vi "Button_handling.vi"(7 "connect":bool, 10 "Z_HSwitch":bool, 11 "Z_Source":T2=enum."local disabled") -> (3 "Z_HSwitch_state":T1={"Write"=FALSE, "Z1_ind"=5, "Z1_ind_blinking"=FALSE, "Z_HSwitch_out"=FALSE, "Z_HSwitch_visible"=FALSE, "Z_HSwitch_disabled"=enum."Enabled"})   [LabVIEW 2019]
uses:
  Y_source.ctl
  OLD/Button state.ctl
  Timer Delay/Timers.lvlib
panel:
  out "Z1 ind":u8(ring)
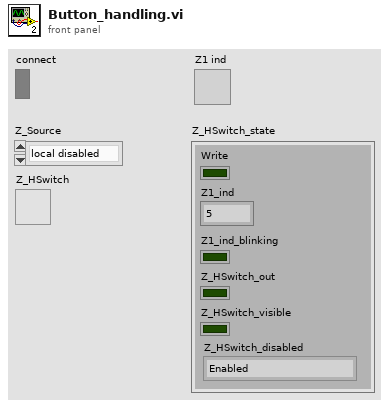
[diagram p1: front panel]
types:
  T1 = cluster{"Write":bool, "Z1_ind":u8, "Z1_ind_blinking":bool, "Z_HSwitch_out":bool, "Z_HSwitch_visible":bool, "Z_HSwitch_disabled":enum8{"Enabled", "Disabled", "Disabled and Grayed Out"}}
  T2 = typedef "Y_source.ctl" = enum8{"initialize", "local disabled", "local hand", "hand", "auto", "dist"}
  T3 = enum8{"Enabled", "Disabled", "Disabled and Grayed Out"}
  T4 = typedef "Button state.ctl" = enum16{"init", "not connect", "local disabled", "local hand", "set hand", "hand", "set auto", "auto", "dist"}
  T5 = cluster{"Write":bool, "Z1_ind visu":u8, "Z1_ind_blinking":bool, "Z_HSwitch_out":bool, "Z_HSwitch_visible":bool, "Z_HSwitch_disabled":enum8{"Enabled", "Disabled", "Disabled and Grayed Out"}}
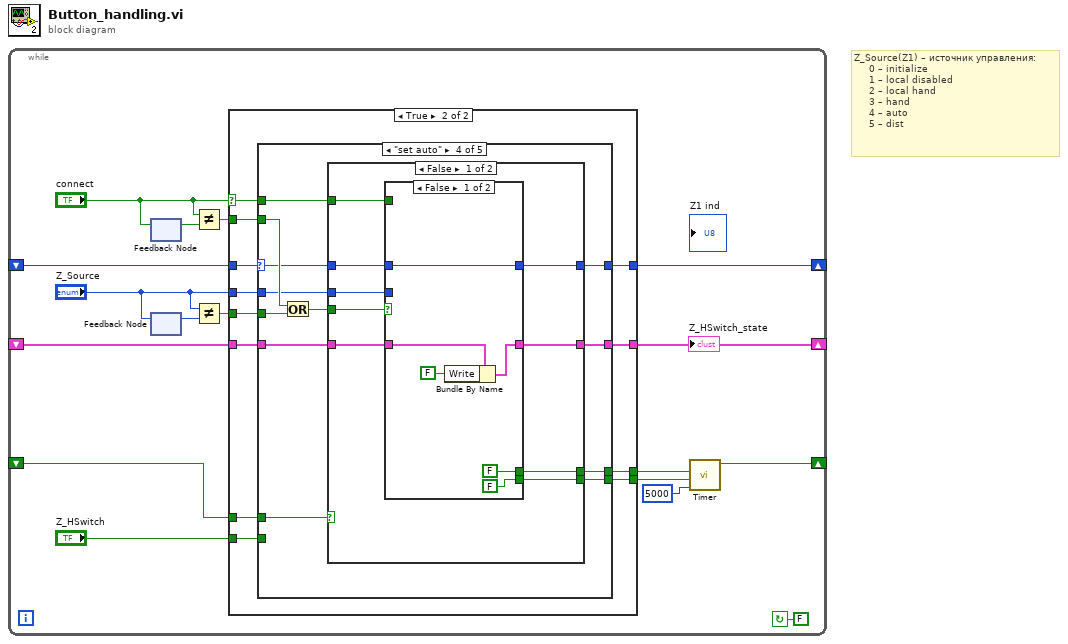
[diagram p0: block diagram]
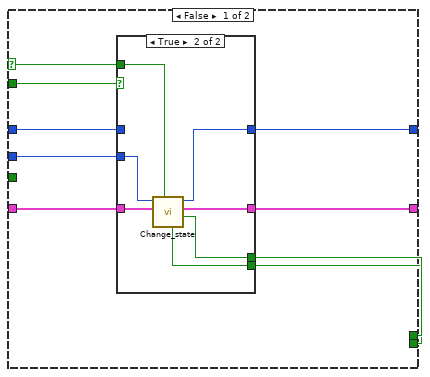
[diagram p2: hidden frame]
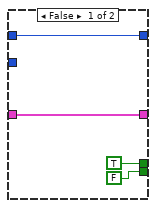
[diagram p3: hidden frame]
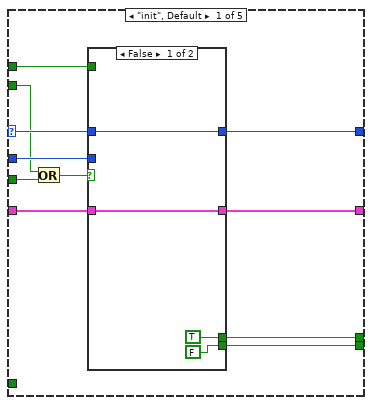
[diagram p4: hidden frame]
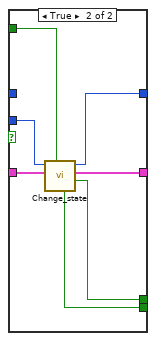
[diagram p5: hidden frame]
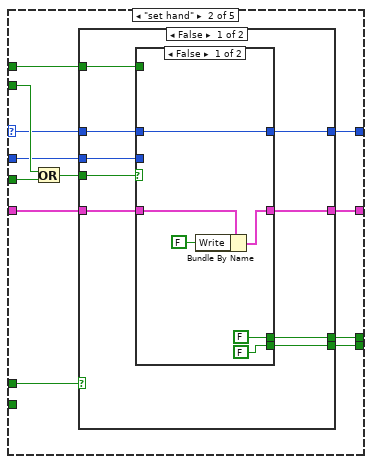
[diagram p6: hidden frame]
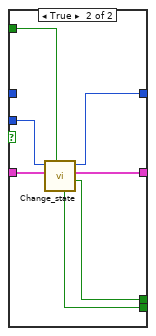
[diagram p7: hidden frame]
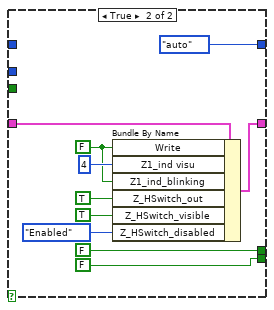
[diagram p8: hidden frame]
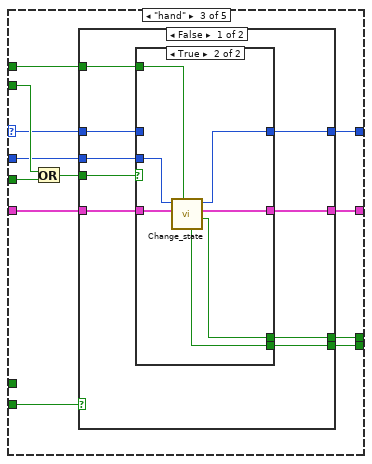
[diagram p9: hidden frame]
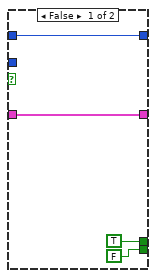
[diagram p10: hidden frame]
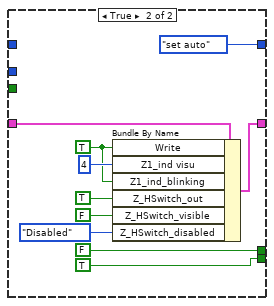
[diagram p11: hidden frame]
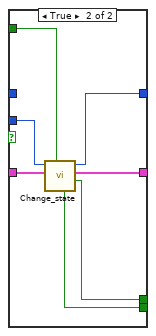
[diagram p12: hidden frame]
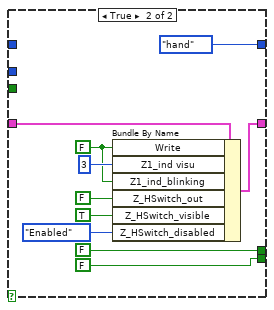
[diagram p13: hidden frame]
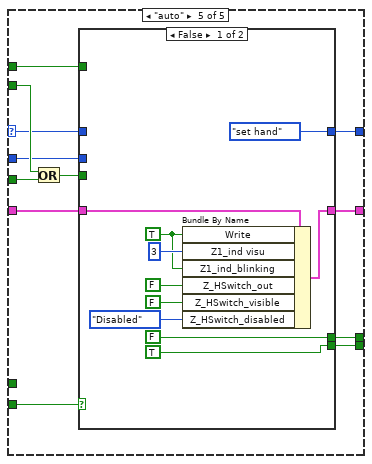
[diagram p14: hidden frame]
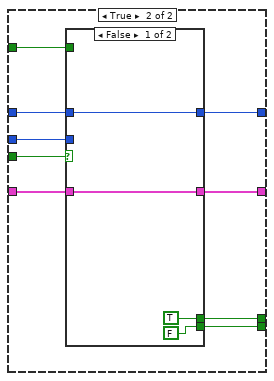
[diagram p15: hidden frame]
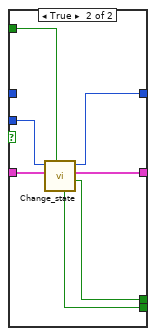
[diagram p16: hidden frame]
diagram:
  # "Z_Source(Z1) – источник управления:\n     0 – initialize\n     1 – local disabled\n     2 – local hand\n     3 – hand\n     4 – аuto\n     5 – dist"
  n1 = while {
    shift-right: [w17] -> _
    shift-left: _ -> [w1]
    shift-right: [w12] -> _
    shift-left: _ -> [w16]
    shift-right: [w10] -> _
    shift-left: _ -> [w13]
    stop <- FALSE continue-if-true
    n2 = feedback #1() -> (w4:bool)  [unwired: 1 in]
    n3 = feedback-in #1("connect") -> ()
    n4 = feedback #2() -> (w7:T2)  [unwired: 1 in]
    n5 = feedback-in #2("Z_Source") -> ()
    n6 = Not Equal?(x="connect", y=w4) -> (x != y?=w2:bool)
    n7 = Not Equal?(x="Z_Source", y=w7) -> (x != y?=w5:bool)
    n8 = case shown="True" "connect" {
      selector: "connect" -> [w18 w40]
      tunnel: [w23 w49] -> w17
      tunnel: w16 -> [_ w48]
      tunnel: w13 -> [w24 w47]
      tunnel: w1 -> [w26 w46]
      tunnel: "Z_HSwitch" -> [_ w45]
      tunnel: "Z_Source" -> [w25 w44]
      tunnel: [w22 w43] -> w10
      tunnel: [w21 w42] -> w9
      tunnel: [w20 w41] -> w8
      tunnel: w5 -> [_ w39]
      tunnel: w2 -> [w19 w38]
      frame False {
        n9 = case shown="True" w19 {
          tunnel: w24 -> [w30 w37]
          tunnel: [w30 w36] -> w22
          tunnel: [TRUE ("reset_timer") w35] -> w21
          tunnel: [FALSE ("load_timer") w34] -> w20
          tunnel: [w27 w33] -> w23
          tunnel: w25 -> [_ w32]
          tunnel: w26 -> [w27 _]
          tunnel: w18 -> [_ w31]
          frame False {
          }
          frame True {
            n10 = call "Change_state.vi"("connect (T)"=w31, "Z_HSwitch_state in"=w37, "Z_Source"=w32) -> ("reset_timer"=w35:bool, "Z_HSwitch_state out"=w36:T5, "Z1_ind_state"=w33:T4, "load_timer"=w34:bool)  [unwired: 5 in]
          }
        }
      }
      frame True {
        n11 = case shown="\"set auto\"" w46 {
          selector: w46 -> [w54 w75 w119 w161 w205]
          tunnel: w45 -> [_ _ w121 _ w207]
          tunnel: [w55 w81 w125 w167 w211] -> w49
          tunnel: w44 -> [w59 w74 w118 w160 w204]
          tunnel: w48 -> [_ w77 _ w163 _]
          tunnel: [w58 w79 w123 w165 w209] -> w42
          tunnel: [w57 w78 w122 w164 w208] -> w41
          tunnel: [w56 w80 w124 w166 w210] -> w43
          tunnel: w47 -> [w60 w72 w116 w158 w202]
          tunnel: w40 -> [w51 w76 w120 w162 w206]
          tunnel: w39 -> [w52 w82 w126 w168 w212]
          tunnel: w38 -> [w50 w83 w127 w169 w213]
          frame "init", Default {
            # "local hand"
            n12 = Or(x=w50, y=w52) -> (x .or. y?=w53:bool)
            n13 = case shown="False" w53 {
              tunnel: w60 -> [w64 w71]
              tunnel: [w64 w70] -> w56
              tunnel: [TRUE ("reset_timer") w69] -> w58
              tunnel: [FALSE ("load_timer") w68] -> w57
              tunnel: [w61 w67] -> w55
              tunnel: w59 -> [_ w66]
              tunnel: w51 -> [_ w65]
              tunnel: w54 -> [w61 _]
              frame False {
              }
              frame True {
                n14 = call "Change_state.vi"("connect (T)"=w65, "Z_HSwitch_state in"=w71, "Z_Source"=w66) -> ("reset_timer"=w69:bool, "Z_HSwitch_state out"=w70:T5, "Z1_ind_state"=w67:T4, "load_timer"=w68:bool)  [unwired: 5 in]
              }
            }
          }
          frame "set hand" {
            # "local hand"
            n15 = Or(x=w83, y=w82) -> (x .or. y?=w73:bool)
            n16 = case shown="False" w77 {
              tunnel: w75 -> [w87 _]
              tunnel: [w86 Button_state."auto" ("f 3")] -> w81
              tunnel: [w84 w110] -> w80
              tunnel: w72 -> [w85 w109]
              tunnel: [w89 FALSE ("Z_ASwitch")] -> w79
              tunnel: [w88 FALSE ("Z_ASwitch")] -> w78
              tunnel: w76 -> [w92 _]
              tunnel: w74 -> [w91 _]
              tunnel: w73 -> [w90 _]
              frame False {
                n17 = case shown="False" w90 {
                  tunnel: w85 -> [w94 w105]
                  tunnel: [w93 w104] -> w84
                  tunnel: [FALSE ("reset_timer") w103] -> w89
                  tunnel: [FALSE ("load_timer") w102] -> w88
                  tunnel: [w96 w101] -> w86
                  tunnel: w91 -> [_ w100]
                  tunnel: w92 -> [_ w99]
                  tunnel: w87 -> [w96 _]
                  frame False {
                    n18 = Bundle By Name(cluster=w94, "Write"=FALSE) -> (w93:T5)
                  }
                  frame True {
                    n19 = call "Change_state.vi"("connect (T)"=w99, "Z_HSwitch_state in"=w105, "Z_Source"=w100) -> ("reset_timer"=w103:bool, "Z_HSwitch_state out"=w104:T5, "Z1_ind_state"=w101:T4, "load_timer"=w102:bool)  [unwired: 5 in]
                  }
                }
              }
              frame True {
                w112 = FALSE ("Z_ASwitch")
                n20 = Bundle By Name(cluster=w109, "Write"=w112, "Z1_ind visu"=u8 4, "Z1_ind_blinking"=w112, "Z_HSwitch_out"=TRUE ("Z_ASwitch"), "Z_HSwitch_visible"=TRUE ("Z_ASwitch"), "Z_HSwitch_disabled"=T3."Enabled" ("Disabled")) -> (w110:T5)
              }
            }
          }
          frame "hand" {
            # "local hand"
            n21 = Or(x=w127, y=w126) -> (x .or. y?=w117:bool)
            n22 = case shown="False" w121 {
              tunnel: w119 -> [w129 _]
              tunnel: [w128 Button_state."set auto" ("f 3")] -> w125
              tunnel: [w130 w152] -> w124
              tunnel: w116 -> [w131 w151]
              tunnel: [w133 FALSE ("Z_ASwitch")] -> w123
              tunnel: [w132 TRUE ("Z_ASwitch")] -> w122
              tunnel: w120 -> [w136 _]
              tunnel: w118 -> [w135 _]
              tunnel: w117 -> [w134 _]
              frame False {
                n23 = case shown="True" w134 {
                  tunnel: w131 -> [w140 w147]
                  tunnel: [w140 w146] -> w130
                  tunnel: [TRUE ("reset_timer") w145] -> w133
                  tunnel: [FALSE ("load_timer") w144] -> w132
                  tunnel: [w137 w143] -> w128
                  tunnel: w135 -> [_ w142]
                  tunnel: w136 -> [_ w141]
                  tunnel: w129 -> [w137 _]
                  frame False {
                  }
                  frame True {
                    n24 = call "Change_state.vi"("connect (T)"=w141, "Z_HSwitch_state in"=w147, "Z_Source"=w142) -> ("reset_timer"=w145:bool, "Z_HSwitch_state out"=w146:T5, "Z1_ind_state"=w143:T4, "load_timer"=w144:bool)  [unwired: 5 in]
                  }
                }
              }
              frame True {
                w154 = TRUE ("Z_ASwitch")
                n25 = Bundle By Name(cluster=w151, "Write"=w154, "Z1_ind visu"=u8 4, "Z1_ind_blinking"=w154, "Z_HSwitch_out"=TRUE ("Z_ASwitch"), "Z_HSwitch_visible"=FALSE ("Z_ASwitch"), "Z_HSwitch_disabled"=T3."Disabled" ("Disabled")) -> (w152:T5)
              }
            }
          }
          frame "set auto" {
            # "local hand"
            n26 = Or(x=w169, y=w168) -> (x .or. y?=w159:bool)
            n27 = case shown="False" w163 {
              tunnel: w161 -> [w173 _]
              tunnel: [w172 Button_state."hand" ("f 3")] -> w167
              tunnel: [w170 w196] -> w166
              tunnel: w158 -> [w171 w195]
              tunnel: [w175 FALSE ("Z_ASwitch")] -> w165
              tunnel: [w174 FALSE ("Z_ASwitch")] -> w164
              tunnel: w162 -> [w178 _]
              tunnel: w160 -> [w177 _]
              tunnel: w159 -> [w176 _]
              frame False {
                n28 = case shown="False" w176 {
                  tunnel: w171 -> [w180 w191]
                  tunnel: [w179 w190] -> w170
                  tunnel: [FALSE ("reset_timer") w189] -> w175
                  tunnel: [FALSE ("load_timer") w188] -> w174
                  tunnel: [w182 w187] -> w172
                  tunnel: w177 -> [_ w186]
                  tunnel: w178 -> [_ w185]
                  tunnel: w173 -> [w182 _]
                  frame False {
                    n29 = Bundle By Name(cluster=w180, "Write"=FALSE) -> (w179:T5)
                  }
                  frame True {
                    n30 = call "Change_state.vi"("connect (T)"=w185, "Z_HSwitch_state in"=w191, "Z_Source"=w186) -> ("reset_timer"=w189:bool, "Z_HSwitch_state out"=w190:T5, "Z1_ind_state"=w187:T4, "load_timer"=w188:bool)  [unwired: 5 in]
                  }
                }
              }
              frame True {
                w198 = FALSE ("Z_ASwitch")
                n31 = Bundle By Name(cluster=w195, "Write"=w198, "Z1_ind visu"=u8 3, "Z1_ind_blinking"=w198, "Z_HSwitch_out"=FALSE ("Z_ASwitch"), "Z_HSwitch_visible"=TRUE ("Z_ASwitch"), "Z_HSwitch_disabled"=T3."Enabled" ("Disabled")) -> (w196:T5)
              }
            }
          }
          frame "auto" {
            # "local hand"
            n32 = Or(x=w213, y=w212) -> (x .or. y?=w203:bool)
            n33 = case shown="False" w207 {
              tunnel: w205 -> [_ w225]
              tunnel: [Button_state."set hand" ("f 3") w224] -> w211
              tunnel: [w218 w226] -> w210
              tunnel: w202 -> [w217 w227]
              tunnel: [FALSE ("Z_ASwitch") w229] -> w209
              tunnel: [TRUE ("Z_ASwitch") w228] -> w208
              tunnel: w206 -> [_ w232]
              tunnel: w204 -> [_ w231]
              tunnel: w203 -> [_ w230]
              frame False {
                w220 = TRUE ("Z_ASwitch")
                n34 = Bundle By Name(cluster=w217, "Write"=w220, "Z1_ind visu"=u8 3, "Z1_ind_blinking"=w220, "Z_HSwitch_out"=FALSE ("Z_ASwitch"), "Z_HSwitch_visible"=FALSE ("Z_ASwitch"), "Z_HSwitch_disabled"=T3."Disabled" ("Disabled")) -> (w218:T5)
              }
              frame True {
                n35 = case shown="False" w230 {
                  tunnel: w227 -> [w236 w243]
                  tunnel: [w236 w242] -> w226
                  tunnel: [TRUE ("reset_timer") w241] -> w229
                  tunnel: [FALSE ("load_timer") w240] -> w228
                  tunnel: [w233 w239] -> w224
                  tunnel: w231 -> [_ w238]
                  tunnel: w232 -> [_ w237]
                  tunnel: w225 -> [w233 _]
                  frame False {
                  }
                  frame True {
                    n36 = call "Change_state.vi"("connect (T)"=w237, "Z_HSwitch_state in"=w243, "Z_Source"=w238) -> ("reset_timer"=w241:bool, "Z_HSwitch_state out"=w242:T5, "Z1_ind_state"=w239:T4, "load_timer"=w240:bool)  [unwired: 5 in]
                  }
                }
              }
            }
          }
        }
      }
    }
    "Z_HSwitch_state" <- w10
    n37 = call "Timer.vi"("ms"=5000, "Load (F)"=w8, "Reset (F)"=w9) -> ("End"=w12:bool)  [unwired: 6 in, 1 out]
  }
